vi "map_to_array_buffer.vi"(8 "error in (no error)":errorcluster, 10 "Pixel block":sgl[](array[numeric]), 11 "ImageAssemblerRK110612Spiral in":refnum<class "ImageAssemblerRK110612Spiral.lvclass">) -> (0 "error out":errorcluster, 3 "ImageAssemblerRK110612Spiral out":refnum<class "ImageAssemblerRK110612Spiral.lvclass">)   [LabVIEW 2010, in "ImageAssemblerRK110612Spiral.lvclass"]
uses:
  ImageAssemblerRK110612Spiral.lvclass
  ImageAssemblerRK110612Spiral.lvclass/ImageAssemblerRK110612Spiral.ctl
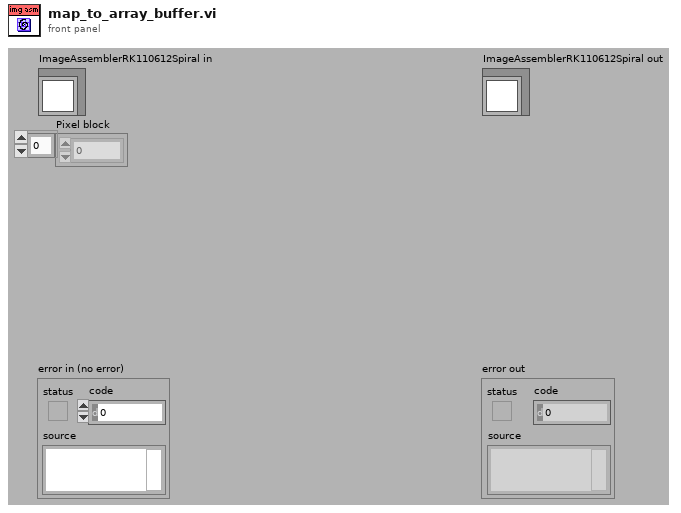
[diagram p1: front panel]
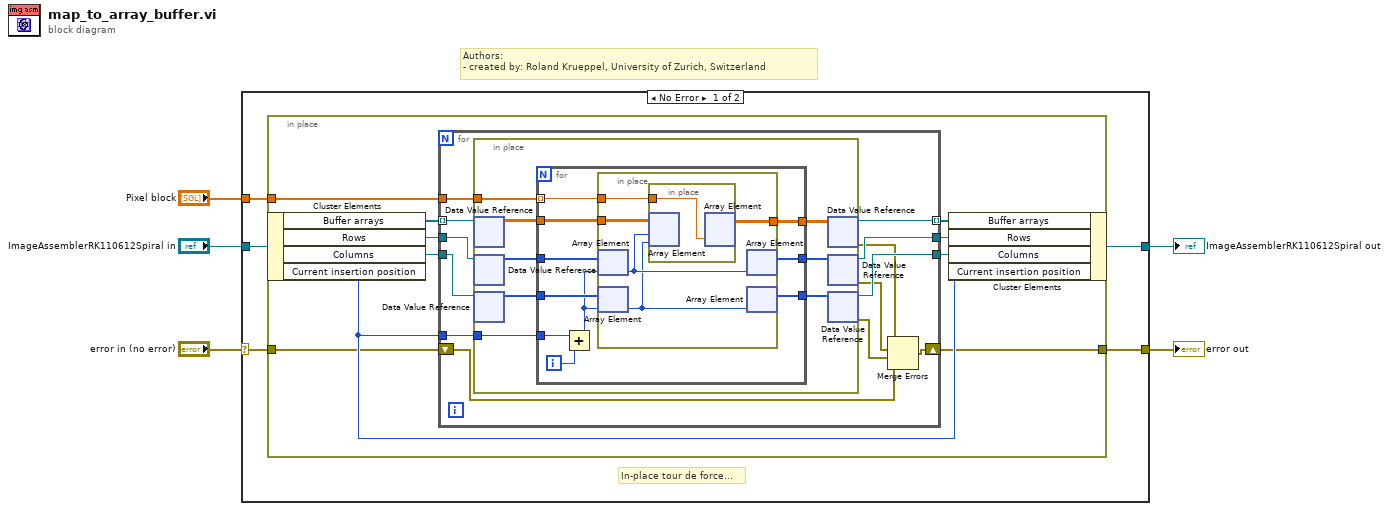
[diagram p0: block diagram]
diagram:
  # "Authors: \n- created by: Roland Krueppel, University of Zurich, Switzerland"
  n1 = case shown="No Error" "error in (no error)" {
    selector: "error in (no error)" -> [w7 w59]
    tunnel: [w6 w59] -> w4
    tunnel: [w9 w58] -> w2
    tunnel: "ImageAssemblerRK110612Spiral in" -> [w10 w58]
    tunnel: "Pixel block" -> [w8 _]
    frame No Error {
      # "In-place tour de force..."
      n2 = in-place {
        in-place-border: w8 -> [w18]
        in-place-border: w7 -> [w12]
        in-place-border: [w11] -> w6
        n3 = in-place-cluster #1(w10) -> ("Buffer arrays"=w17:refnum<data-value>[], "Rows"=w20:refnum<data-value>, "Columns"=w19:refnum<data-value>, "Current insertion position"=w14:i32)
        n4 = for {
          tunnel: w20 -> [w33]
          tunnel: w19 -> [w32]
          tunnel: w18 -> [w31]
          tunnel: w17 -> [w30] mode=indexing
          tunnel: [w29] -> w16 mode=indexing
          tunnel: [w28] -> w15
          tunnel: [w27] -> w13
          tunnel: w14 -> [w26]
          shift-right: [w22] -> w11
          shift-left: w12 -> [w21]
          n5 = in-place {
            in-place-border: w31 -> [w41]
            in-place-border: w26 -> [w38]
            n6 = in-place-dvr #2(w30) -> (w35:sgl[][])  [unwired: 1 out]
            n7 = in-place-dvr #3(w33) -> (w40:i32[])  [unwired: 1 out]
            n8 = in-place-dvr #4(w32) -> (w39:i32[])  [unwired: 1 out]
            n9 = for {
              tunnel: w41 -> [w43] mode=indexing
              tunnel: w40 -> [w51]
              tunnel: w39 -> [w50]
              tunnel: w38 -> [w49]
              tunnel: [w46] -> w37
              tunnel: [w45] -> w36
              tunnel: w35 -> [w44]
              tunnel: [w42] -> w34
              i -> [w48]
              n10 = Add(x=w49, y=w48) -> (x+y=w47:i32)
              n11 = in-place {
                in-place-border: w44 -> [w56]
                in-place-border: w43 -> [w53]
                in-place-border: [w52] -> w42
                n12 = in-place-array #5(w51, w47) -> (w55:i32)
                n13 = in-place-array #6(w50, w47) -> (w54:i32)
                n14 = in-place {
                  in-place-border: w53 -> [w57]
                  n15 = in-place-array #7(w56, w55, w54) -> ()  [unwired: 1 out]
                  n16 = in-place-array #7(w57) -> (w52:sgl[][])  [unwired: 2 out]
                }
                n17 = in-place-array #5(w55) -> (w46:i32[])  [unwired: 1 out]
                n18 = in-place-array #6(w54) -> (w45:i32[])  [unwired: 1 out]
              }
            }
            n19 = in-place-dvr #2(w34) -> (w29:refnum<data-value>, w25:errorcluster)
            n20 = in-place-dvr #3(w37) -> (w28:refnum<data-value>, w24:errorcluster)
            n21 = in-place-dvr #4(w36) -> (w27:refnum<data-value>, w23:errorcluster)
          }
          n22 = Merge Errors(w25, w24, w23, w21) -> (w22:errorcluster)
        }
        n23 = in-place-cluster #1("Buffer arrays"=w16, "Rows"=w15, "Columns"=w13, "Current insertion position"=w14) -> (w9:refnum<class "ImageAssemblerRK110612Spiral.lvclass">)
      }
    }
    frame Error {
    }
  }
  "error out" <- w4
  "ImageAssemblerRK110612Spiral out" <- w2
